vi "Disconnect Core.vi"(8 "error in (no error)":errorcluster, 10 "Force (T)":bool=TRUE, 11 "PVConnection in":refnum<class "DSConnection.lvclass">) -> (0 "error out":errorcluster, 3 "PVConnection out":refnum<class "DSConnection.lvclass">)   [LabVIEW 2016, in "CS++ProcessVariables.lvlib" / "DSConnection.lvclass"]
doc: "Close reference to a process variable."
uses:
  DSConnection.lvclass
  DSConnection.lvclass/DSConnection.ctl
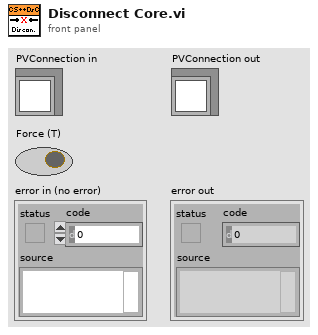
[diagram p1: front panel]
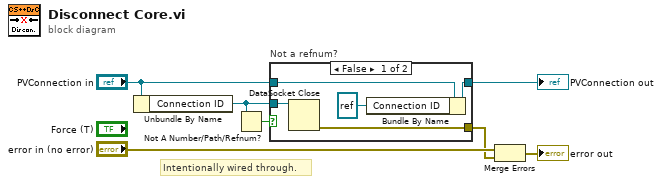
[diagram p0: block diagram]
diagram:
  # "Intentionally wired through."
  n1 = Unbundle By Name("PVConnection in") -> ("Connection ID"=w5:refnum<k13>)
  n2 = Not A Number/Path/Refnum?(number/path/refnum=w5) -> (NaN/Path/Refnum?=w4:bool)
  n3 = case "Not a refnum?" shown="False" w4 {
    tunnel: w5 -> [w12 _]
    tunnel: [w11 _] -> w1
    tunnel: "PVConnection in" -> [w10 w13]
    tunnel: [w9 w13] -> w6
    frame False {
      n4 = DataSocket Close(11:w12) -> (0:w11:errorcluster)  [unwired: 2 in, 1 out]
      n5 = Bundle By Name(cluster=w10, "Connection ID"=refnum<k13> refnum) -> (w9:refnum<class "DSConnection.lvclass">)
    }
    frame True {
    }
  }
  "PVConnection out" <- w6
  n6 = Merge Errors("error in (no error)", w1) -> (→"error out":errorcluster)
